vi "Select SubPanel.vi"(8 "error in (no error)":errorcluster, 10 "Arguments":string, 11 "UI.Lockin":refnum<class "UI.Lockin.lvclass">) -> (0 "error out":errorcluster, 2 "UI_":refnum<class "Instrument UI.lvclass">, 3 "UI.Lockin out":refnum<class "UI.Lockin.lvclass">)   [LabVIEW 2019, in "UI.Lockin.lvclass"]
uses:
  UI.Lockin.lvclass
  UI_DAQ_config/UI.Lockin.DAQ_config.lvclass
  C:/Program Files (x86)/National Instruments/LabVIEW 2019/user.lib/LevyLab/Instrument Framework/SMOs/Instrument UI/Instrument UI.lvclass
  C:/Program Files (x86)/National Instruments/LabVIEW 2019/vi.lib/JKI/JKI SMO/SMO.UI/SMO.UI.lvclass
  C:/Program Files (x86)/National Instruments/LabVIEW 2019/vi.lib/JKI/JKI SMO/SMO/SMO.lvclass
  UI_DSP_Config/UI.Lockin.DSP_Config.lvclass
  UI_Generator_Config/UI.Lockin.Generator_Config.lvclass
  UI_Scope/UI.Lockin.Scope.lvclass
  <userlib>/LevyLab/Instrument Framework/SMOs/Instrument UI/Instrument UI.lvclass
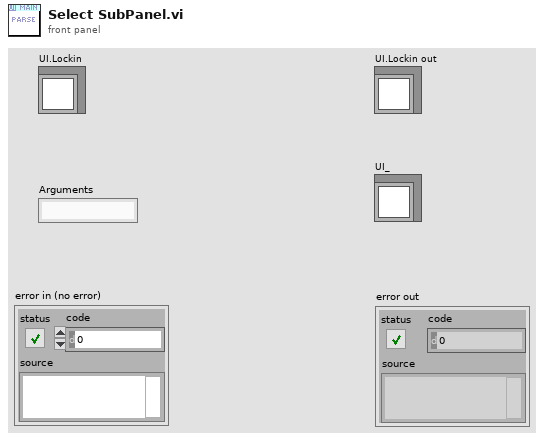
[diagram p1: front panel]
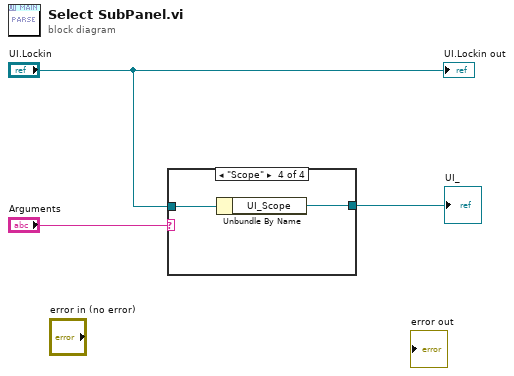
[diagram p0: block diagram]
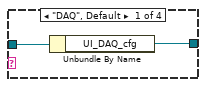
[diagram p2: hidden frame]
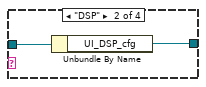
[diagram p3: hidden frame]
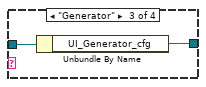
[diagram p4: hidden frame]
diagram:
  n1 = case shown="\"Scope\"" "Arguments" {
    tunnel: [w5 w7 w9 w11] -> w1
    tunnel: "UI.Lockin" -> [w4 w6 w8 w10]
    frame "DAQ", Default {
      n2 = Unbundle By Name(w4) -> ("UI_DAQ_cfg"=w5:refnum<class "UI.Lockin.DAQ_config.lvclass">)
    }
    frame "DSP" {
      n3 = Unbundle By Name(w6) -> ("UI_DSP_cfg"=w7:refnum<class "UI.Lockin.DSP_Config.lvclass">)
    }
    frame "Generator" {
      n4 = Unbundle By Name(w8) -> ("UI_Generator_cfg"=w9:refnum<class "UI.Lockin.Generator_Config.lvclass">)
    }
    frame "Scope" {
      n5 = Unbundle By Name(w10) -> ("UI_Scope"=w11:refnum<class "UI.Lockin.Scope.lvclass">)
    }
  }
  "UI_" <- w1
  "UI.Lockin out" <- "UI.Lockin"
